vi "U6 Line-to-Line.vi"() -> ()   [LabVIEW 2021]
panel:
  in  "Pulse Width [ms]":u32=500
  in  "DeviceType":u16(ring)=1 items=["LJ_dtU3", "LJ_dtU6", "LJ_dtUE9"]
  out "10k Ticks":u32
  out "Period [s]":dbl format="%.6f"
  in  "error in":errorcluster
  in  "ConnectionType":u16(ring) items=["LJ_ctUSB", "LJ_ctETHERNET"]
  in  "Address":string="1"
  in  "FirstFound":bool=TRUE
  out "error out":errorcluster
  out "Error Message":string
  # "Enables line-to-line timer mode on FIO0 and FIO1.  FIO0 starts the counting on a rising edge,\nand FIO1 stops the counting on the next falling edge.  Clock is set to 1M/100 => 10 kHz, so\neach tick corresponds to 100us and the 16-bit counter can count up to 6.5535 seconds.\n\nFIO3 is used to create an output pulse using a simple software delay."
  # "Input"
  # "Output"
  # "6500 max to prevent\n16-bit value from\nrolling."
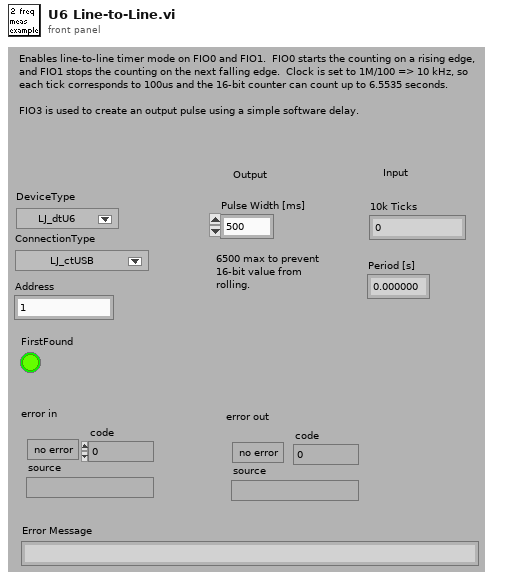
[diagram p1: front panel]
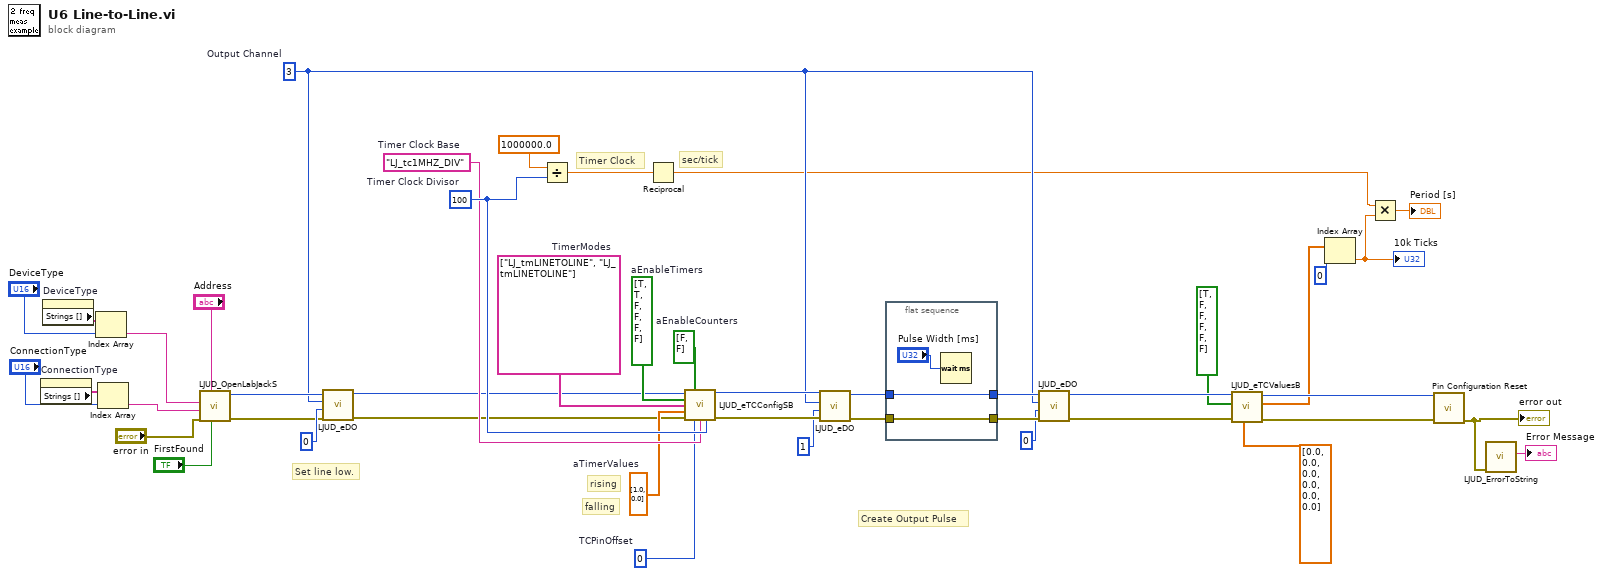
[diagram p0: block diagram]
diagram:
  w8 = 3  # Output Channel
  w23 = dbl[] [1.0, 0.0]  # aTimerValues
  w24 = 0  # TCPinOffset
  w29 = bool[] [FALSE, FALSE]  # aEnableCounters
  w30 = bool[] [TRUE, TRUE, FALSE, FALSE, FALSE, FALSE]  # aEnableTimers
  w32 = 100  # Timer Clock Divisor
  w31 = "LJ_tc1MHZ_DIV"  # Timer Clock Base
  w33 = string[] ["LJ_tmLINETOLINE", "LJ_tmLINETOLINE"]  # TimerModes
  # "Create Output Pulse"
  # "Set line low."
  # "falling"
  # "rising"
  # "Timer Clock"
  # "sec/tick"
  n1 = property on="ConnectionType" class="Ring (strict)"() -> ("Strings []"=w38:string[])  [unwired: 2 in, 2 out]
  n2 = property on="DeviceType" class="Ring (strict)"() -> ("Strings []"=w39:string[])  [unwired: 2 in, 2 out]
  n3 = Index Array(array=w39, index="DeviceType") -> (element=w34:string)
  n4 = Index Array(array=w38, index="ConnectionType") -> (element=w35:string)
  n5 = call "LJUD_OpenLabJackS.vi"("FirstFound"="FirstFound", "Address"="Address", "error in"="error in", "ConnectionType"=w35, "DeviceType"=w34) -> ("error out"=w19:errorcluster, "Handle"=w21:i32)  [unwired: 4 in, 1 out]
  n6 = call "LJUD_eDO.vi"("error in"=w19, "State"=0, "Channel"=w8, "Handle In"=w21) -> ("error out"=w18:errorcluster, "Handle Out"=w20:i32)  [unwired: 6 in]
  n7 = Divide(x=1000000.0, y=w32) -> (x/y=w40:dbl)
  n8 = Reciprocal(x=w40) -> (1/x=w3:dbl)
  n9 = call "LJUD_eTCConfigSB.vi"("Handle In"=w20, "aEnableCounters"=w29, "aEnableTimers"=w30, "aTimerModes"=w33, "aTimerValues"=w23, "error in"=w18, "TCPinOffset"=w24, "TimerClockBase"=w31, "TimerClockDivisor"=w32) -> ("Handle Out"=w13:i32, "error out"=w17:errorcluster)  [unwired: 5 in]
  n10 = call "LJUD_eDO.vi"("error in"=w17, "State"=1, "Channel"=w8, "Handle In"=w13) -> ("error out"=w16:errorcluster, "Handle Out"=w12:i32)  [unwired: 6 in]
  n11 = flat-sequence {
    tunnel: w16 -> [w48]
    tunnel: [w48] -> w15
    tunnel: w12 -> [w47]
    tunnel: [w47] -> w11
    frame #0 {
      n12 = Wait (ms)(milliseconds to wait="Pulse Width [ms]") -> ()  [unwired: 1 out]
    }
  }
  n13 = call "LJUD_eDO.vi"("error in"=w15, "State"=0, "Channel"=w8, "Handle In"=w11) -> ("error out"=w14:errorcluster, "Handle Out"=w10:i32)  [unwired: 6 in]
  n14 = call "LJUD_eTCValuesB.vi"("aTimerValues Write"=dbl[] [0.0, 0.0, 0.0, 0.0, 0.0, 0.0] ("TimerValues"), "error in"=w14, "aReadTimers"=bool[] [TRUE, FALSE, FALSE, FALSE, FALSE, FALSE] ("UpdateReset Timers"), "Handle In"=w10) -> ("error out"=w27:errorcluster, "aTimerValues Read"=w6:dbl[], "Handle Out"=w28:i32)  [unwired: 4 in, 1 out]
  n15 = Index Array(array=w6, index=0) -> (element=w4:dbl)
  "10k Ticks" <- w4
  n16 = Multiply(x=w3, y=w4) -> (x*y=→"Period [s]":dbl)
  n17 = call "Pin Configuration Reset.vi"("error in"=w27, "Handle In"=w28) -> ("error out"=w26:errorcluster)  [unwired: 8 in, 1 out]
  "error out" <- w26
  n18 = call "LJUD_ErrorToString.vi"("error in"=w26) -> ("String"=→"Error Message":string)  [unwired: 10 in]
